vi "dvp Vi Get Sharpness State.vi"(10 "pSharpnessState":i32, 11 "handle":u32) -> (2 "pSharpnessState out":i32, 3 "function return":u32(ring))   [LabVIEW 2018, in "LabViewDVPCamera.lvlib"]
doc: "LabviewDvp2Api dvpStatus dvpViGetSharpnessState(dvpHandle handle, BOOL *pSharpnessState);"
uses:
  LabViewDVPCamera.lvlib
  LabViewDVPCamera/LabViewDVPCamera.dll
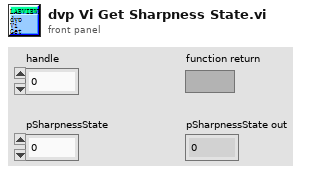
[diagram p1: front panel]
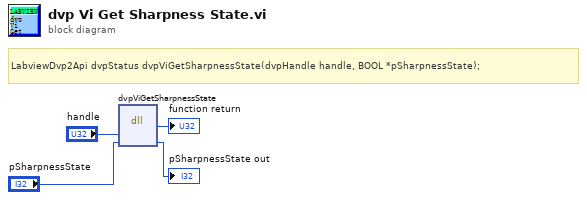
[diagram p0: block diagram]
diagram:
  # "LabviewDvp2Api dvpStatus dvpViGetSharpnessState(dvpHandle handle, BOOL *pSharpnessState);"
  n1 = dll-call lib="C:/Program Files (x86)/DVP2 Labview cn 64/Sample/LabViewDVPCamera/LabViewDVPCamera.*" fn="dvpViGetSharpnessState"("handle"="handle", "pSharpnessState"="pSharpnessState") -> (→"function return":u32, "pSharpnessState"=→"pSharpnessState out":i32)  [unwired: 4 in, 2 out]
